vi "Get Session Properties List.vi"(0 "SLSC Remote in":refnum<class "SLSC Remote.lvclass">, 11 "error in (no error)":errorcluster) -> (4 "SLSC Remote out":refnum<class "SLSC Remote.lvclass">, 8 "Sys.SessionProperties":refnum<k21>[](array[refnum]), 15 "error out":errorcluster)   [LabVIEW 2016, in "SLSC Interfaces.lvlib" / "SLSC Remote.lvclass"]
uses:
  SLSC Remote.lvclass
  C:/Users/tblair/Documents/Git Projects/SLSC-Interface/Source/SLSC Interface Class/SLSC Interface.lvclass
  <vilib>/NI/JSON Support for LabVIEW/JSON Data Classes/JSON Object/JSON Object.lvclass
  C:/Program Files (x86)/National Instruments/LabVIEW 2016/vi.lib/NI/JSON Support for LabVIEW/JSON Data Classes/JSON Datatype/JSON Null.lvclass
  <vilib>/NI/JSON Support for LabVIEW/JSON Data Classes/JSON Object/New JSON Object (Empty).vi
  <vilib>/NI/JSON Support for LabVIEW/JSON Data Classes/JSON Object/Insert Key Value Pair (Single String).vi
  <vilib>/NI/NI JSONRPC Server Framework/Classes/Server/Format Client Request (Auto-Increment).vi
  <vilib>/httpClient/POSTBuffer.vi
  <vilib>/NI/NI JSONRPC Server Framework/Classes/Server/Parse Response (Object).vi
  <vilib>/NI/JSON Support for LabVIEW/JSON Data Classes/JSON Object/Get Value (Array).vi
  <vilib>/NI/JSON Support for LabVIEW/JSON Data Classes/JSON Array/Index Array (String Value).vi
  <vilib>/NI/NI JSONRPC Server Framework/Classes/Server/JSONRPC Server.lvclass
  <vilib>/httpClient/LabVIEWHTTPClient.lvlib
  <vilib>/NI/JSON Support for LabVIEW/JSON Data Classes/JSON Helper/JSON Helper.lvclass
  <vilib>/NI/JSON Support for LabVIEW/JSON Data Classes/JSON Array/JSON Array.lvclass
  C:/Program Files (x86)/National Instruments/LabVIEW 2016/vi.lib/NI/JSON Support for LabVIEW/JSON Data Classes/JSON Structured Type/JSON Structure.lvclass
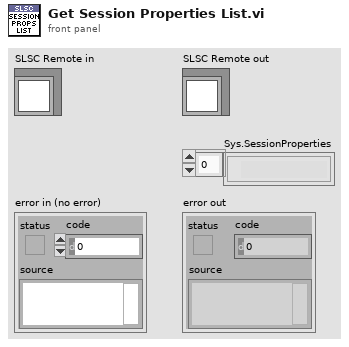
[diagram p1: front panel]
types:
  T1 = typedef "LabVIEWHTTPClient.lvlib/ClientHandle.ctl" = refnum<k1>
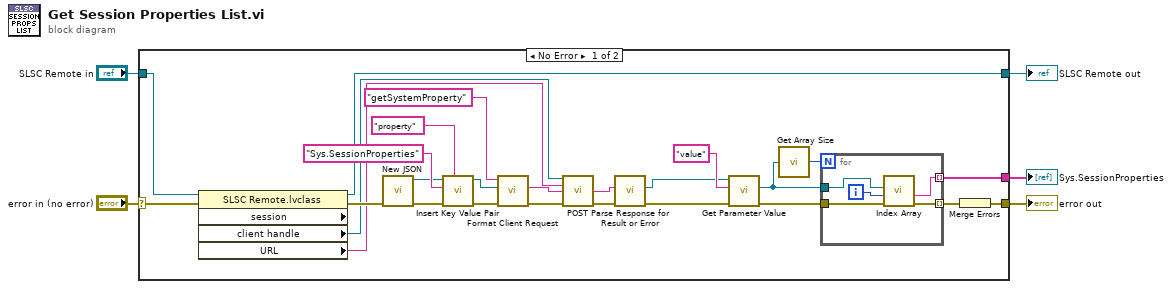
[diagram p0: block diagram]
diagram:
  n1 = case shown="No Error" "error in (no error)" {
    selector: "error in (no error)" -> [w29 w37]
    tunnel: "SLSC Remote in" -> [w31 w38]
    tunnel: [w30 w38] -> w3
    tunnel: [w10 w37] -> w2
    tunnel: [w11 _] -> w1
    frame No Error {
      n2 = property class="SLSC Remote.lvclass" props=["session", "client handle", "URL"](reference=w31, error in=w29) -> (reference out=w30:refnum<class "SLSC Remote.lvclass">, error out=w28:errorcluster, "client handle"=w24:T1, "URL"=w23:string)  [unwired: 1 out]
      n3 = call-poly <vilib>:"New JSON.vi"("error in (no error)"=w28) -> ("error out"=w27:errorcluster, "JSON Object out"=w7:refnum<class "JSON Object.lvclass">)  [unwired: 9 in]
      n4 = call-poly <vilib>:"Insert Key Value Pair.vi"("key"="property" ("Name"), "error in (no error)"=w27, "value"="Sys.SessionProperties" ("String"), "JSON Object in"=w7) -> ("error out"=w18:errorcluster, "JSON Object out"=w19:refnum<class "JSON Object.lvclass">)  [unwired: 5 in, 1 out]
      n5 = call-poly <vilib>:"Format Client Request.vi"("error in (no error)"=w18, "JSON in"=w19, "method"="getSystemProperty") -> ("error out"=w22:errorcluster, "Request String"=w25:string)  [unwired: 7 in]
      n6 = call-poly <vilib>:"POST.vi"("client handle"=w24, "url"=w23, "buffer"=w25, "error in (no error)"=w22) -> ("body"=w21:string, "error out"=w20:errorcluster)  [unwired: 8 in, 2 out]
      n7 = call-poly <vilib>:"Parse Response for Result or Error.vi"("error in"=w20, "Response String In"=w21) -> ("error out"=w16:errorcluster, "JSON Array"=w6:refnum<class "JSON Object.lvclass">)  [unwired: 7 in, 1 out]
      n8 = call-poly <vilib>:"Get Parameter Value.vi"("error in (no error)"=w16, "key"="value" ("Parameter Name"), "JSON Object in"=w6) -> ("error out"=w13:errorcluster, "value"=w14:refnum<class "JSON Array.lvclass">)  [unwired: 7 in]
      n9 = call <vilib>:"Get Array Size.vi"("JSON Array in"=w14) -> ("size(s)"=w15:i32)
      n10 = for {
        N: w15 -> [_]
        tunnel: w14 -> [w35]
        tunnel: w13 -> [w34]
        tunnel: [w33] -> w12 mode=indexing
        tunnel: [w32] -> w11 mode=indexing
        i -> [w36]
        n11 = call-poly <vilib>:"Index Array.vi"("error in (no error)"=w34, "index"=w36, "JSON Array in"=w35) -> ("error out"=w33:errorcluster, "String"=w32:string)  [unwired: 7 in]
      }
      n12 = Merge Errors(w12) -> (w10:errorcluster)
    }
    frame Error {
    }
  }
  "error out" <- w2
  "SLSC Remote out" <- w3
  "Sys.SessionProperties" <- w1
